vi "Find_Node_index.vi"(4 "Node Array out":cluster{"Address":i16, "Serial Number":i8[]}[](array[cluster]) {"Serial Number" format="%.0x"; "Address" format="%.0x"}, 5 "Node adress":u16 format="%.0x") -> (0 "Node found":bool, 1 "Message":string, 2 "Node index":i32)   [LabVIEW 2017]
doc: "This VI searches in 'Node array' for a CAN node with an adress specified in 'Node adress'.\nIf it is found 'Node found' is set to TRUE and an ASCII string text message is returned.\nThe place in the 'Node array' is returned in 'Node index'.\nThis VI does not communicate with any I/O device."
panel:
  # "Find which Node index to use with a particular node adress.\nChristian Holmstedt 2002-06-24."
  # "Node Address"
  # "Serial Number"
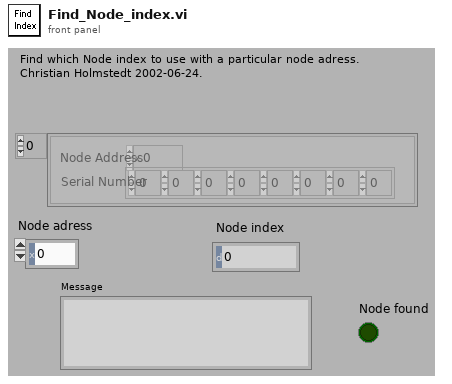
[diagram p1: front panel]
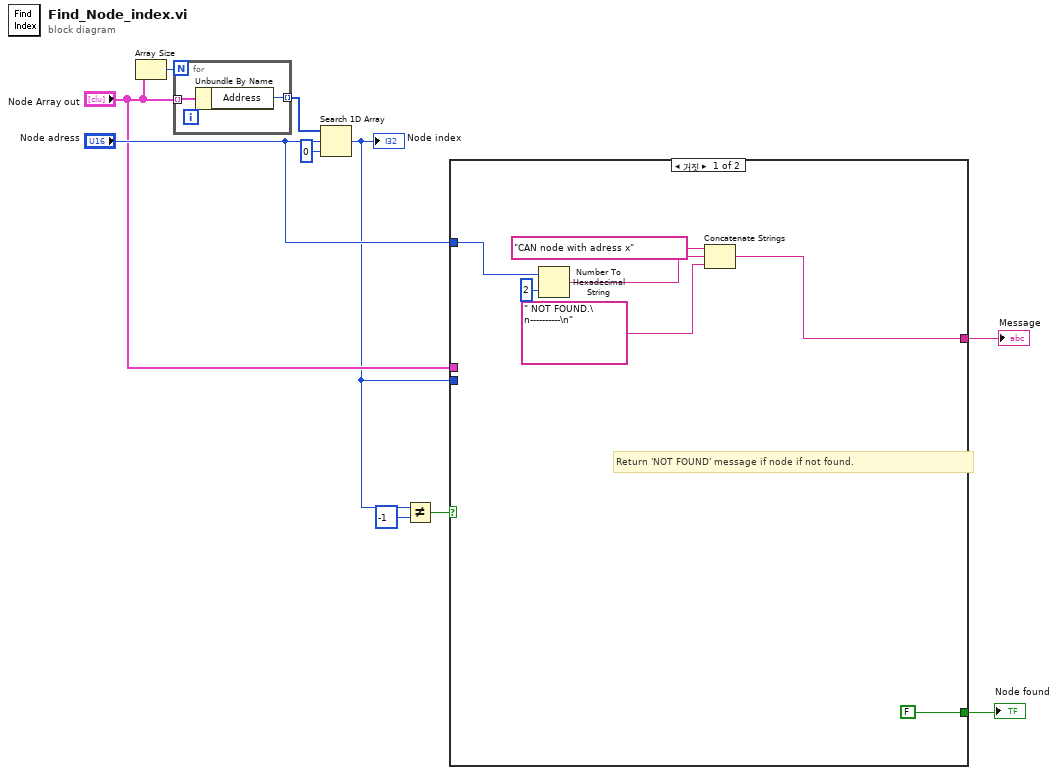
[diagram p0: block diagram]
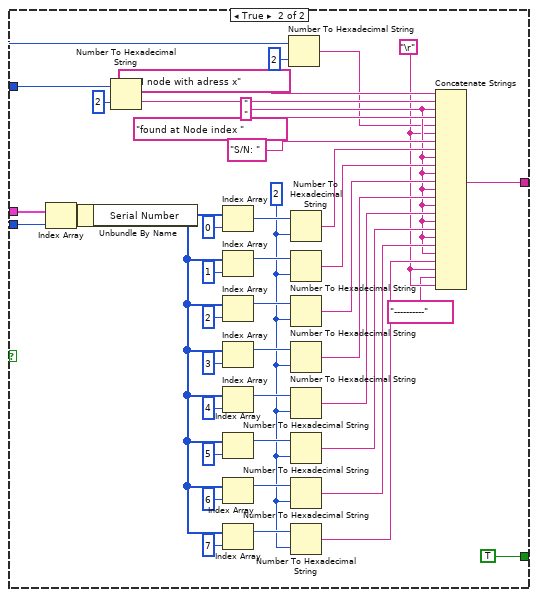
[diagram p2: hidden frame]
diagram:
  n1 = Array Size(array="Node Array out") -> (size(s)=w10:i32)
  n2 = for {
    N: w10 -> [_]
    tunnel: "Node Array out" -> [w12] mode=indexing
    tunnel: [w11] -> w9 mode=indexing
    n3 = Unbundle By Name(w12) -> ("Address"=w11:i16)
  }
  n4 = Search 1D Array(1D array=w9, element="Node adress", start index (0)=0) -> (index of element=w3:i32)
  "Node index" <- w3
  n5 = Not Equal?(x=w3, y=-1) -> (x != y?=w4:bool)
  n6 = case shown="거짓" w4 {
    tunnel: "Node adress" -> [w16 w61]
    tunnel: "Node Array out" -> [_ w55]
    tunnel: [w13 w26] -> w5
    tunnel: w3 -> [_ w25]
    tunnel: [FALSE TRUE] -> w1
    frame False {
      # "Return 'NOT FOUND' message if node if not found."
      n7 = Number To Hexadecimal String(1:i16 2 ("width (-)"), 2:w16) -> (0:w15:string)
      n8 = Concatenate Strings("CAN node with adress x", w15, " NOT FOUND.\n----------\n") -> (w13:string)
    }
    frame True {
      w36 = i16 2 ("width (-)")
      w22 = "\r"
      w28 = " " ("Substring")
      n9 = Index Array(array=w55, index=w25) -> (element=w54:cluster{"Address":i16, "Serial Number":i8[]})
      n10 = Unbundle By Name(w54) -> ("Serial Number"=w53:i8[])
      n11 = Number To Hexadecimal String(1:i16 2 ("width (-)"), 2:w61) -> (0:w58:string)
      n12 = Index Array(array=w53, index=0 ("Index")) -> (element=w44:i8)
      n13 = Index Array(array=w53, index=1 ("Index")) -> (element=w43:i8)
      n14 = Index Array(array=w53, index=2 ("Index")) -> (element=w42:i8)
      n15 = Index Array(array=w53, index=3 ("Index")) -> (element=w41:i8)
      n16 = Index Array(array=w53, index=4 ("Index")) -> (element=w40:i8)
      n17 = Index Array(array=w53, index=5 ("Index")) -> (element=w39:i8)
      n18 = Index Array(array=w53, index=6 ("Index")) -> (element=w38:i8)
      n19 = Index Array(array=w53, index=7 ("Index")) -> (element=w37:i8)
      n20 = Number To Hexadecimal String(1:i16 2 ("width (-)"), 2:w25) -> (0:w23:string)
      n21 = Number To Hexadecimal String(1:w36, 2:w44) -> (0:w35:string)
      n22 = Number To Hexadecimal String(1:w36, 2:w43) -> (0:w34:string)
      n23 = Number To Hexadecimal String(1:w36, 2:w42) -> (0:w33:string)
      n24 = Number To Hexadecimal String(1:w36, 2:w41) -> (0:w32:string)
      n25 = Number To Hexadecimal String(1:w36, 2:w40) -> (0:w31:string)
      n26 = Number To Hexadecimal String(1:w36, 2:w39) -> (0:w30:string)
      n27 = Number To Hexadecimal String(1:w36, 2:w38) -> (0:w29:string)
      n28 = Number To Hexadecimal String(1:w36, 2:w37) -> (0:w27:string)
      n29 = Concatenate Strings("CAN node with adress x", w58, w28, "found at Node index ", w23, w22, "S/N: ", w35, w28, w34, w28, w33, w28, w32, w28, w31, w28, w30, w28, w29, w28, w27, w22, "----------", w22) -> (w26:string)
    }
  }
  "Message" <- w5
  "Node found" <- w1
